vi "PayExtra.vi"() -> ()   [LabVIEW 2023]
panel:
  out "concatenated string":string
  out "date/time string":string
  in  "parked when?":string caption="godzina zaparkowania"
  in  "Error In":errorcluster
  in  "payed":string caption="na ile opłacono"
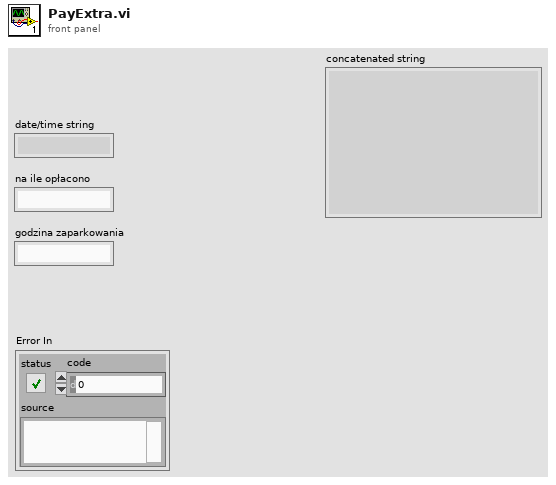
[diagram p1: front panel]
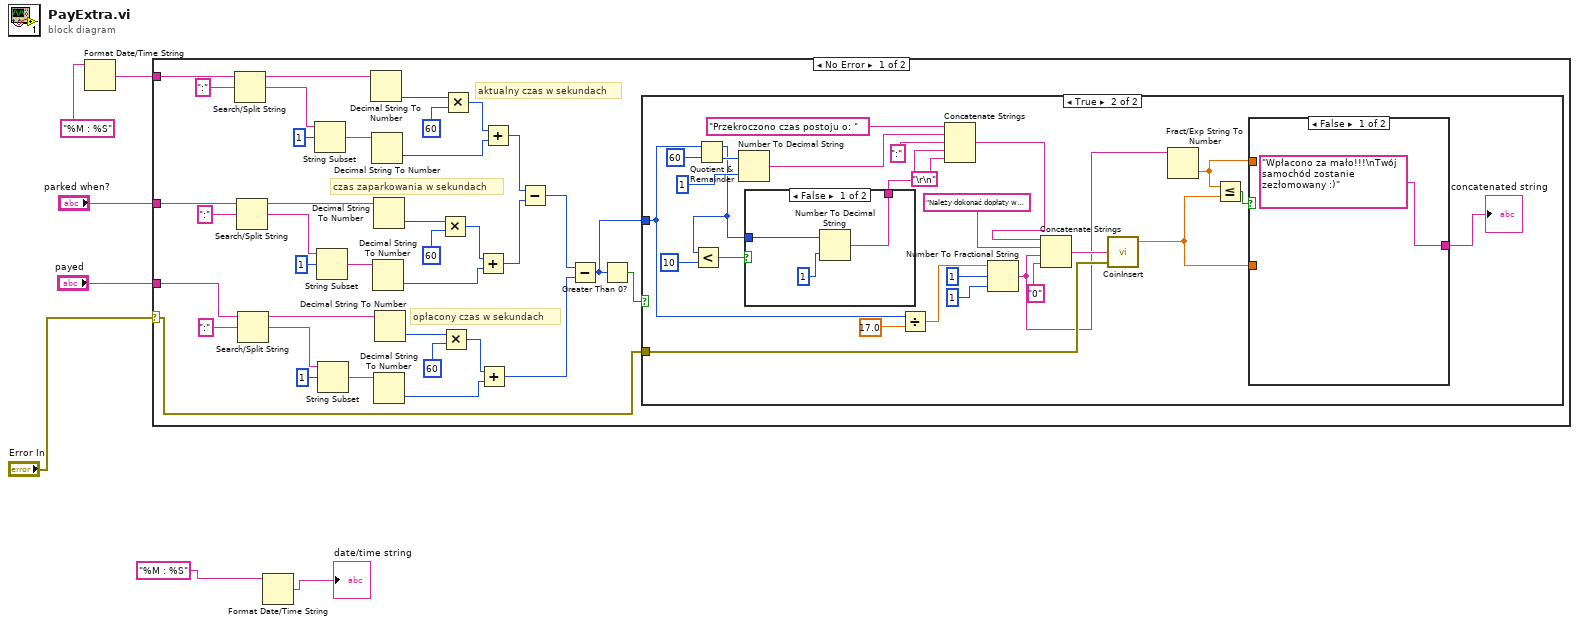
[diagram p0: block diagram]
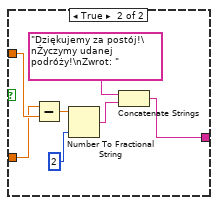
[diagram p3: hidden frame]
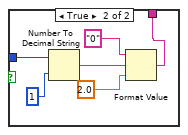
[diagram p4: hidden frame]
diagram:
  n1 = Format Date/Time String(time format string (%c)="%M : %S") -> (date/time string=w3:string)  [unwired: 2 in]
  n2 = case shown="No Error" "Error In" {
    selector: "Error In" -> [w8 _]
    tunnel: "parked when?" -> [w44 _]
    tunnel: w3 -> [w37 _]
    tunnel: "payed" -> [w13 _]
    frame No Error {
      # "opłacony czas w sekundach"
      # "czas zaparkowania w sekundach"
      # "aktualny czas w sekundach"
      n3 = Search/Split String(string=w37, search string/char (-)=":") -> (substring before match=w34:string, match + rest of string=w40:string)  [unwired: 1 in, 1 out]
      n4 = Search/Split String(string=w44, search string/char (-)=":") -> (substring before match=w36:string, match + rest of string=w42:string)  [unwired: 1 in, 1 out]
      n5 = Search/Split String(string=w13, search string/char (-)=":") -> (substring before match=w19:string, match + rest of string=w21:string)  [unwired: 1 in, 1 out]
      n6 = String Subset(string=w40, offset (0)=1) -> (substring=w33:string)  [unwired: 1 in]
      n7 = String Subset(string=w42, offset (0)=1) -> (substring=w35:string)  [unwired: 1 in]
      n8 = String Subset(string=w21, offset (0)=1) -> (substring=w18:string)  [unwired: 1 in]
      n9 = Decimal String To Number(string=w34) -> (number=w26:i32)  [unwired: 2 in, 1 out]
      n10 = Decimal String To Number(string=w33) -> (number=w25:i32)  [unwired: 2 in, 1 out]
      n11 = Decimal String To Number(string=w35) -> (number=w29:i32)  [unwired: 2 in, 1 out]
      n12 = Decimal String To Number(string=w36) -> (number=w32:i32)  [unwired: 2 in, 1 out]
      n13 = Decimal String To Number(string=w18) -> (number=w14:i32)  [unwired: 2 in, 1 out]
      n14 = Decimal String To Number(string=w19) -> (number=w17:i32)  [unwired: 2 in, 1 out]
      n15 = Multiply(x=w32, y=60) -> (x*y=w30:i32)
      n16 = Multiply(x=w17, y=60) -> (x*y=w15:i32)
      n17 = Multiply(x=w26, y=60) -> (x*y=w27:i32)
      n18 = Add(x=w30, y=w29) -> (x+y=w23:i32)
      n19 = Add(x=w15, y=w14) -> (x+y=w11:i32)
      n20 = Add(x=w27, y=w25) -> (x+y=w24:i32)
      n21 = Subtract(x=w24, y=w23) -> (x-y=w12:i32)
      n22 = Subtract(x=w12, y=w11) -> (x-y=w9:i32)
      n23 = Greater Than 0?(x=w9) -> (x > 0?=w10:bool)
      n24 = case shown="True" w10 {
        tunnel: w9 -> [_ w57]
        tunnel: w8 -> [_ w50]
        frame False {
        }
        frame True {
          n25 = Quotient & Remainder(x=w57, y=60) -> (x-y*floor(x/y)=w60:i32, floor(x/y)=w68:i32)
          n26 = Less?(x=w60, y=10) -> (x < y?=w64:bool)
          n27 = Number To Decimal String(number=w68, width (-)=i16 1) -> (decimal integer string=w66:string)
          n28 = case shown="False" w64 {
            tunnel: [w80 w83] -> w62
            tunnel: w60 -> [w79 w82]
            frame False {
              n29 = Number To Decimal String(number=w79, width (-)=i16 1) -> (decimal integer string=w80:string)
            }
            frame True {
              n30 = Number To Decimal String(number=w82, width (-)=i16 1) -> (decimal integer string=w84:string)
              n31 = Format Value(string ("")="0", format string=w84, value (0)=2.0) -> (output string=w83:string)
            }
          }
          n32 = Divide(x=w57, y=17.0) -> (x/y=w55:dbl)
          n33 = Concatenate Strings("Przekroczono czas postoju o: ", w66, ":" ("string"), w62, "\r\n") -> (w59:string)
          n34 = Number To Fractional String(number=w55, width (-)=i16 1, precision (6)=i16 1) -> (F-format string=w49:string)  [unwired: 1 in]
          n35 = Concatenate Strings(w59, "Należy dokonać dopłaty w wysokości: " ("string"), w49, "0" ("string")) -> (w51:string)
          n36 = call "CoinInsert.vi"("Error In"=w50, "InfoIn"=w51) -> ("tyle siana"=w46:dbl)  [unwired: 1 in, 2 out]
          n37 = Fract/Exp String To Number(string=w49) -> (number=w47:dbl)  [unwired: 3 in, 1 out]
          n38 = Less Or Equal?(x=w47, y=w46) -> (x <= y?=w48:bool)
          n39 = case shown="False" w48 {
            tunnel: w47 -> [_ w74]
            tunnel: w46 -> [_ w73]
            tunnel: ["Wpłacono za mało!!!\nTwój samochód zostanie zezłomowany :)" w72] -> w45
            frame False {
            }
            frame True {
              n40 = Subtract(x=w73, y=w74) -> (x-y=w77:dbl)
              n41 = Number To Fractional String(number=w77, precision (6)=i16 2) -> (F-format string=w76:string)  [unwired: 2 in]
              n42 = Concatenate Strings("Dziękujemy za postój!\nŻyczymy udanej podróży!\nZwrot: ", w76) -> (w72:string)
            }
          }
          "concatenated string" <- w45
        }
      }
    }
    frame Error {
    }
  }
  n43 = Format Date/Time String(time format string (%c)="%M : %S") -> (date/time string=→"date/time string":string)  [unwired: 2 in]
